vi "Resolve Arg Path.vi"(9 "index of element":i32, 10 "Custom Parameters":string[](array[string]), 11 "Working Directory":path) -> (3 "Resolved Path":path)   [LabVIEW 2020]
uses:
  <vilib>/LabVIEW Open Source Project/OpenURI/openURI.lvlib
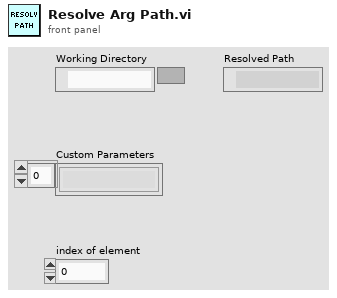
[diagram p1: front panel]
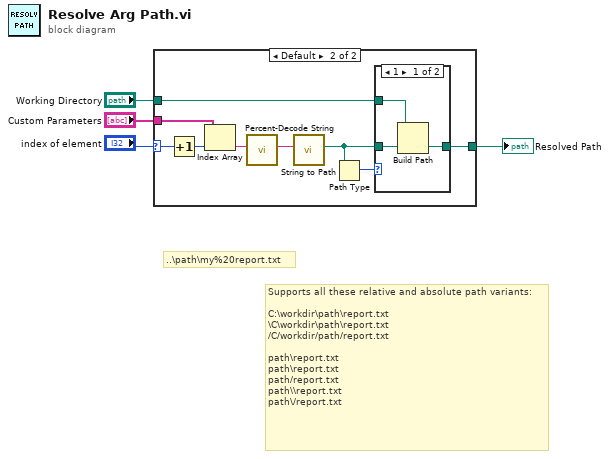
[diagram p0: block diagram]
diagram:
  # "Supports all these relative and absolute path variants:\n\nC:\\workdir\\path\\report.txt\n\\C\\workdir\\path\\report.txt\n/C/workdir/path/report.txt\n\npath\\report.txt\npath\\report.txt\npath/report.txt\npath\\\\report.txt\npath\\/report.txt"
  # "..\\path\\my%20report.txt"
  n1 = case shown="Default" "index of element" {
    selector: "index of element" -> [_ w12]
    tunnel: "Custom Parameters" -> [_ w11]
    tunnel: [_ w8] -> w2
    tunnel: "Working Directory" -> [_ w7]
    frame -1 {
    }
    frame Default {
      n2 = Increment(x=w12) -> (x+1=w13:i32)
      n3 = Index Array(array=w11, index=w13) -> (element=w10:string)
      n4 = call <vilib>:"Percent-Decode String.vi"("Pct-Encoded String"=w10) -> ("String"=w9:string)  [unwired: 10 in]
      n5 = call <vilib>:"String to Path.vi"("common path"=w9) -> ("Path"=w5:path)  [unwired: 10 in]
      n6 = Path Type(1:w5) -> (0:w6:i16)
      n7 = case shown="1" w6 {
        tunnel: w5 -> [w14 w17]
        tunnel: [w15 w17] -> w8
        tunnel: w7 -> [w16 _]
        frame 1 {
          n8 = Build Path(base path=w16, name or relative path=w14) -> (appended path=w15:path)
        }
        frame Default {
        }
      }
    }
  }
  "Resolved Path" <- w2
